vi "Simple_Number_Comparison.vi"() -> ()   [LabVIEW 2010]
panel:
  in  "stop":bool
  out "Equal?":bool
  in  "Numeric 2":dbl
  in  "Numeric":dbl
  # "Simple Number Comparison\nBen Harris - TSCT"
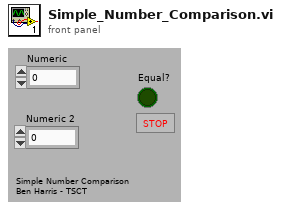
[diagram p1: front panel]
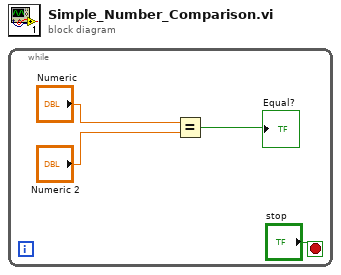
[diagram p0: block diagram]
diagram:
  n1 = while {
    stop <- "stop" stop-if-true
    n2 = Equal?(x="Numeric", y="Numeric 2") -> (x = y?=→"Equal?":bool)
  }
